vi "Minimum_Polynomial_Coefficents.vi"(1 "Calib consts":dbl[](array[numeric]), 2 "Max Length":i32) -> (0 "Coefficients":dbl[](array[numeric]))   [LabVIEW 2011]
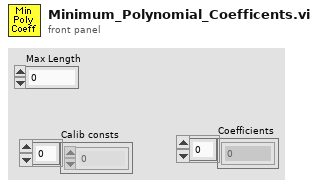
[diagram p1: front panel]
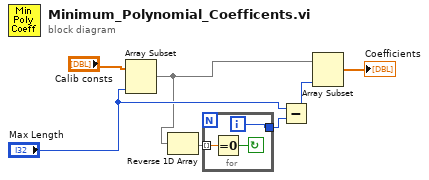
[diagram p0: block diagram]
diagram:
  n1 = Array Subset(array="Calib consts", length="Max Length") -> (w1:dbl[])  [unwired: 1 in]
  n2 = Reverse 1D Array(array=w1) -> (reversed array=w2:dbl[])
  n3 = for {
    tunnel: w2 -> [w10] mode=indexing
    tunnel: [w8] -> w3
    i -> [w8]
    stop <- w9 continue-if-true
    n4 = Equal To 0?(x=w10) -> (x = 0?=w9:bool)
  }
  n5 = Subtract(x="Max Length", y=w3) -> (x-y=w5:i32)
  n6 = Array Subset(array=w1, length=w5) -> (→"Coefficients":dbl[])  [unwired: 1 in]
